vi "waveform_rebin.vi"(5 "Bin size":i16=1, 9 "Waveform Data IN":waveform(dbl)[](graph)=[{"t0"=timestamp(-1.0000000000287557e-06 s since 1904-01-01), "dt"=1e-09, "Y"=array[10001 elements]}]) -> (0 "dt":dbl[](array[numeric]), 1 "Sizes":i32[](array[numeric]), 2 "Waveform Data OUT":waveform(dbl)[](graph)=[{"t0"=timestamp(-1.0000000000287557e-06 s since 1904-01-01), "dt"=1e-09, "Y"=array[10001 elements]}])   [LabVIEW 2015, in "oskar_tools.lvlib"]
uses:
  oskar_tools.lvlib
panel:
  out "Waveform Comparision":waveform(dbl)[](graph)=[{"t0"=timestamp(-1.0000000000287557e-06 s since 1904-01-01), "dt"=1e-09, "Y"=array[10001 elements]}]
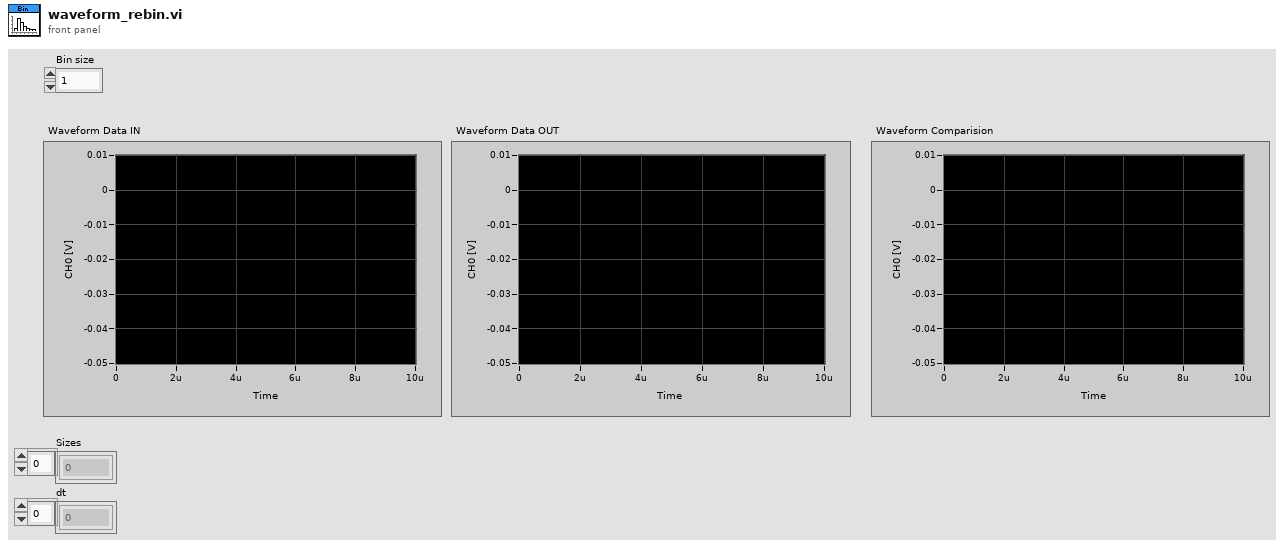
[diagram p1: front panel]
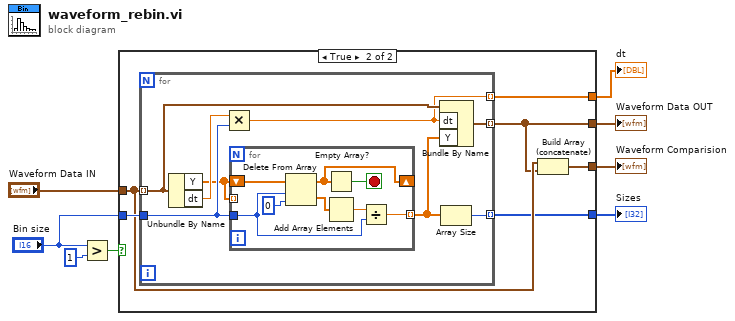
[diagram p0: block diagram]
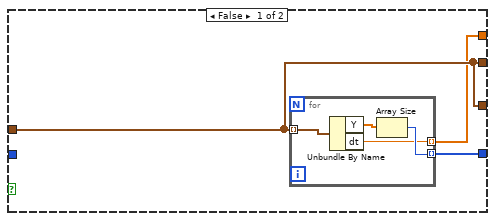
[diagram p2: hidden frame]
diagram:
  n1 = Greater?(x="Bin size", y=i16 1) -> (0:w5:bool)
  n2 = case shown="True" w5 {
    tunnel: "Waveform Data IN" -> [w11 w20]
    tunnel: [w11 w19] -> w7
    tunnel: "Bin size" -> [_ w21]
    tunnel: [w11 w18] -> w3
    tunnel: [w9 w17] -> w2
    tunnel: [w10 w16] -> w1
    frame False {
      n3 = for {
        tunnel: w11 -> [w15] mode=indexing
        tunnel: [w13] -> w10 mode=indexing
        tunnel: [w12] -> w9 mode=indexing
        n4 = Unbundle By Name(w15) -> ("Y"=w14:dbl[], "dt"=w12:dbl)
        n5 = Array Size(array=w14) -> (size(s)=w13:i32)
      }
    }
    frame True {
      n6 = for {
        tunnel: w20 -> [w27] mode=indexing
        tunnel: w21 -> [w28]
        tunnel: [w26] -> w19 mode=indexing
        tunnel: [w23] -> w16 mode=indexing
        tunnel: [w22] -> w17 mode=indexing
        n7 = Unbundle By Name(w27) -> ("Y"=w25:dbl[], "dt"=w29:dbl)
        n8 = Multiply(x=w29, y=w28) -> (x*y=w22:dbl)
        n9 = for {
          shift-right: [w35] -> _
          shift-left: w25 -> [w36]
          tunnel: [w31] -> w24 mode=indexing
          tunnel: w28 -> [w30]
          tunnel: w25 -> [_] mode=indexing
          stop <- w34 stop-if-true
          n10 = Delete From Array(array=w36, length=w30, index=0) -> (deleted portion=w33:dbl[], array with subset deleted=w35:dbl[])
          n11 = Empty Array?(array=w35) -> (empty?=w34:bool)
          n12 = Add Array Elements(numeric array=w33) -> (sum=w32:dbl)
          n13 = Divide(x=w32, y=w30) -> (x/y=w31:dbl)
        }
        n14 = Bundle By Name(cluster=w27, "dt"=w22, "Y"=w24) -> (w26:waveform(dbl))
        n15 = Array Size(array=w24) -> (size(s)=w23:i32)
      }
      n16 = Build Array (concatenate)(w20, w19) -> (w18:waveform(dbl)[])
    }
  }
  "Waveform Data OUT" <- w7
  "Waveform Comparision" <- w3
  "Sizes" <- w1
  "dt" <- w2
